vi "MDTM.vi"(8 "error in (no error)":errorcluster, 10 "RemoteFileName":string, 11 "FTP in":refnum<class "FTP.lvclass">) -> (0 "error out":errorcluster, 2 "Modified Timestamp":timestamp, 3 "FTP out":refnum<class "FTP.lvclass">)   [LabVIEW 2013, in "FTP.lvlib" / "FTP.lvclass"]
uses:
  FTP.lvclass
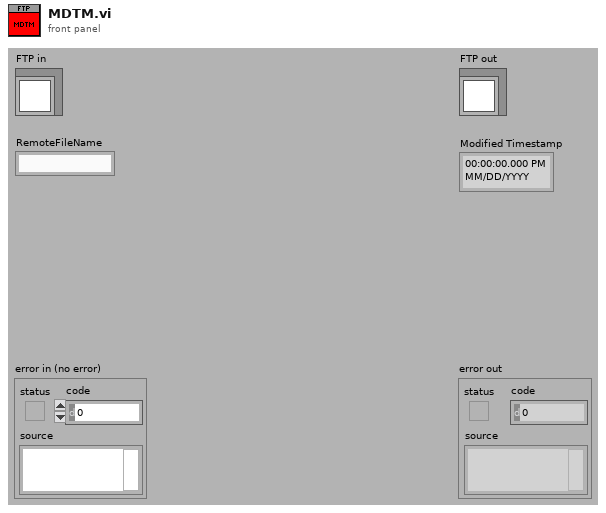
[diagram p1: front panel]
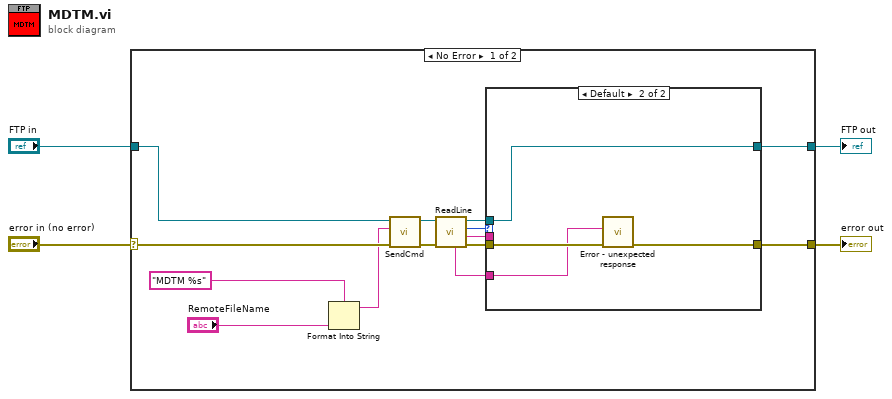
[diagram p0: block diagram]
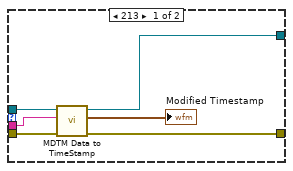
[diagram p2: hidden frame]
diagram:
  n1 = case shown="No Error" "error in (no error)" {
    selector: "error in (no error)" -> [w11 w30]
    tunnel: [w9 w30] -> w3
    tunnel: [w10 w29] -> w1
    tunnel: "FTP in" -> [w12 w29]
    frame No Error {
      n2 = Format Into String(format string="MDTM %s" ("cmd"), "RemoteFileName") -> (resulting string=w7:string)  [unwired: 2 in, 1 out]
      n3 = call "SendCmd.vi"("error in (no error)"=w11, "cmd"=w7, "FTP in"=w12) -> ("error out"=w18:errorcluster, "FTP out"=w17:refnum<class "FTP.lvclass">)  [unwired: 7 in]
      n4 = call "ReadLine.vi"("error in (no error)"=w18, "FTP in"=w17) -> ("error out"=w14:errorcluster, "Line"=w13:string, "code"=w15:i32, "FTP out"=w16:refnum<class "FTP.lvclass">, "Full Line"=w5:string)  [unwired: 5 in]
      n5 = case shown="Default" w15 {
        tunnel: w16 -> [w23 w28]
        tunnel: w14 -> [w24 w27]
        tunnel: [w21 w25] -> w9
        tunnel: [w22 w28] -> w10
        tunnel: w13 -> [w20 _]
        tunnel: w5 -> [_ w26]
        frame 213 {
          n6 = call "MDTM Data to TimeStamp.vi"("error in (no error)"=w24, "MDTM Data"=w20, "FTP in"=w23) -> ("error out"=w21:errorcluster, "time stamp"=→"Modified Timestamp":timestamp, "FTP out"=w22:refnum<class "FTP.lvclass">)  [unwired: 6 in]
        }
        frame Default {
          n7 = call "Error - unexpected response.vi"("error in (no error)"=w27, "Full Response"=w26) -> ("error out"=w25:errorcluster)  [unwired: 9 in]
        }
      }
    }
    frame Error {
    }
  }
  "error out" <- w3
  "FTP out" <- w1
